vi "XML_Node Attributes.vi"(8 "error in":errorcluster caption="错误输入（无错误）", 10 "AttributeNames":string[](array[string])=["Name", "Alias", "ID"], 11 "node in":refnum<k20> caption="节点结果") -> (0 "error out":errorcluster caption="错误输出", 2 "Values":string[](array[string]), 3 "node out":refnum<k20>)   [LabVIEW 2016]
uses:
  <resource>/objmgr/DOMUserDefRef.rc
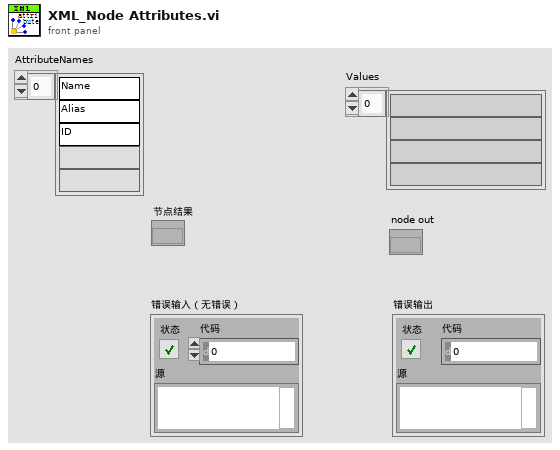
[diagram p1: front panel]
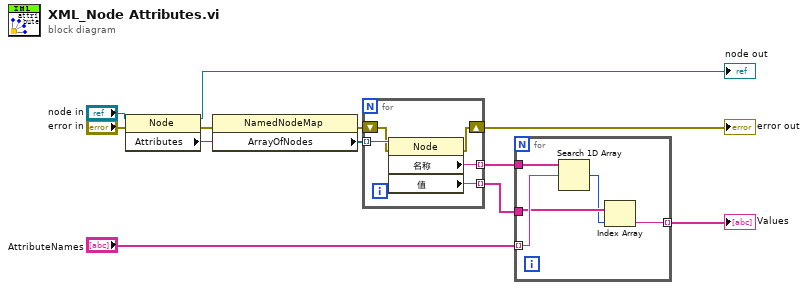
[diagram p0: block diagram]
diagram:
  n1 = property on="属性节点" class="Node"(reference="node in", error in="error in") -> (reference out=→"node out":refnum<k20>, error out=w10:errorcluster, "Attributes"=w12:refnum<k20>)
  n2 = property on="属性节点" class="NamedNodeMap"(reference=w12, error in=w10) -> (error out=w9:errorcluster, "ArrayOfNodes"=w11:refnum<k20>[])  [unwired: 1 out]
  n3 = for {
    tunnel: w11 -> [w17] mode=indexing
    tunnel: [w16] -> w4 mode=indexing
    tunnel: [w15] -> w3 mode=indexing
    shift-right: [w13] -> w6
    shift-left: w9 -> [w14]
    n4 = property on="属性节点" class="Node"(reference=w17, error in=w14) -> (error out=w13:errorcluster, "名称"=w16:string, "值"=w15:string)  [unwired: 1 out]
  }
  "error out" <- w6
  n5 = for {
    tunnel: w4 -> [w22]
    tunnel: w3 -> [w20]
    tunnel: "AttributeNames" -> [w21] mode=indexing
    tunnel: [w18] -> w1 mode=indexing
    n6 = Search 1D Array(1D array=w22, element=w21) -> (index of element=w19:i32)  [unwired: 1 in]
    n7 = Index Array(array=w20, index=w19) -> (element=w18:string)
  }
  "Values" <- w1
